vi "Sub UI Update o point.vi"(8 "error in (no error)":errorcluster, 11 "LF2R IDE in":refnum<class "LF2R IDE.lvclass">) -> (0 "error out":errorcluster, 3 "LF2R IDE out":refnum<class "LF2R IDE.lvclass">)   [LabVIEW 2018, in "LF2R IDE.lvlib" / "LF2R IDE.lvclass"]
uses:
  LF2R IDE.lvclass
  LF2R IDE.lvclass/LF2R IDE.ctl
  Image/Image Process.lvclass
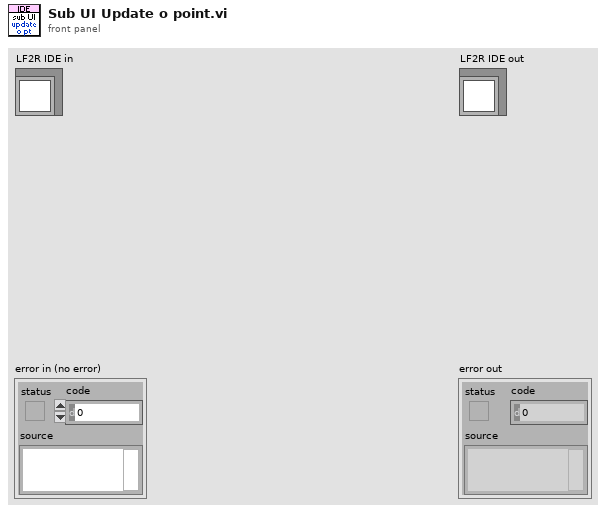
[diagram p1: front panel]
types:
  T1 = typedef "IMAQ Image.ctl" = refnum<image>
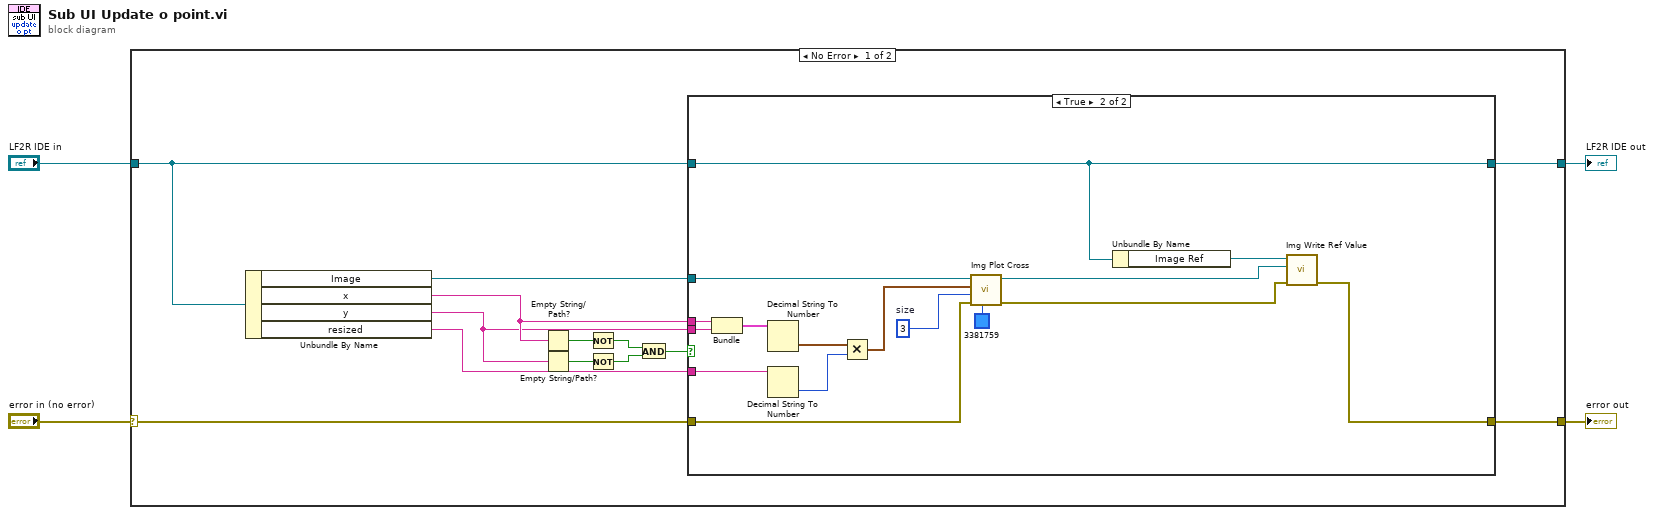
[diagram p0: block diagram]
diagram:
  n1 = case shown="No Error" "error in (no error)" {
    selector: "error in (no error)" -> [w13 w37]
    tunnel: [w16 w37] -> w3
    tunnel: [w5 w36] -> w1
    tunnel: "LF2R IDE in" -> [w17 w36]
    frame No Error {
      n2 = Unbundle By Name(w17) -> ("Image"=w14:T1, "x"=w12:string, "y"=w11:string, "resized"=w15:string)
      n3 = Empty String/Path?(string/path=w12) -> (empty?=w10:bool)
      n4 = Empty String/Path?(string/path=w11) -> (empty?=w9:bool)
      n5 = Not(x=w10) -> (.not. x?=w8:bool)
      n6 = Not(x=w9) -> (.not. x?=w7:bool)
      n7 = And(x=w8, y=w7) -> (x .and. y?=w6:bool)
      n8 = case shown="True" w6 {
        tunnel: w17 -> [w19 w20]
        tunnel: [w18 w34] -> w16
        tunnel: w15 -> [_ w33]
        tunnel: w14 -> [_ w30]
        tunnel: w13 -> [w18 w28]
        tunnel: w12 -> [_ w23]
        tunnel: w11 -> [_ w22]
        tunnel: [w19 w20] -> w5
        frame False {
        }
        frame True {
          w27 = 3  # size
          n9 = Bundle("x"=w23, "y"=w22) -> (w21:cluster{"x":string, "y":string})  [unwired: 1 in]
          n10 = Decimal String To Number(string=w21) -> (number=w32:cluster{"x":i32, "y":i32})  [unwired: 2 in, 1 out]
          n11 = Decimal String To Number(string=w33) -> (number=w31:i32)  [unwired: 2 in, 1 out]
          n12 = Multiply(x=w32, y=w31) -> (x*y=w29:cluster{"x":i32, "y":i32})
          n13 = call "Img Plot Cross.vi"("Color"=u32 3381759, "error in (no error)"=w28, "size"=w27, "position"=w29, "Image In"=w30) -> ("error out"=w25:errorcluster, "Image Out"=w24:T1)  [unwired: 5 in]
          n14 = Unbundle By Name(w20) -> ("Image Ref"=w35:refnum<vi>)
          n15 = call "Img Write Ref Value.vi"("error in (no error)"=w25, "Image"=w24, "Image Ref"=w35) -> ("error out"=w34:errorcluster)  [unwired: 8 in]
        }
      }
    }
    frame Error {
    }
  }
  "error out" <- w3
  "LF2R IDE out" <- w1
